vi "Does the Text Fit.vi"(0 "user-specified font":T1, 5 "token string":string, 7 "Capitalize Text":bool) -> (4 "Text Fits":bool)   [LabVIEW 2020, in "Text-Based VI Icon.lvlib"]
uses:
  <vilib>/LabVIEW Icon API/Set Text Icon/Text-Based VI Icon.lvlib
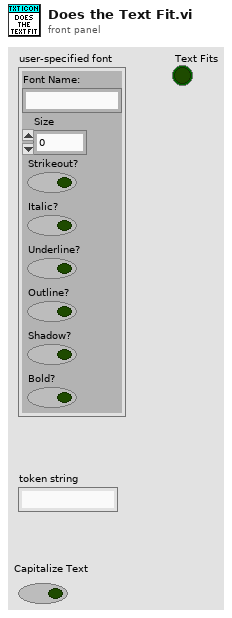
[diagram p1: front panel]
types:
  T1 = cluster{"Font Name:":string, "Size":i16, "Strikeout?":bool, "Italic?":bool, "Underline?":bool, "Outline?":bool, "Shadow?":bool, "Bold?":bool}
  T2 = enum16{"User-specified Font", "Application Font", "System Font", "Dialog Font"}
  T3 = cluster{"left":i16, "top":i16, "right":i16, "bottom":i16}
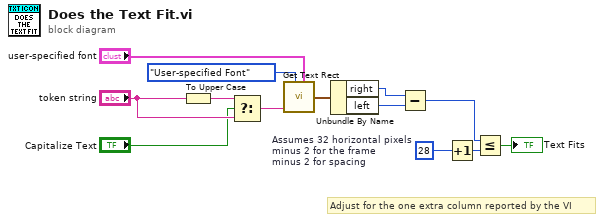
[diagram p0: block diagram]
diagram:
  w9 = i16 28  # Assumes 32 horizontal pixels minus 2 for the frame minus 2 for spacing
  # "Adjust for the one extra column reported by the VI"
  n1 = To Upper Case(1:"token string") -> (0:w4:string)
  n2 = Select(t=w4, s="Capitalize Text", f="token string") -> (s? t:f=w1:string)
  n3 = call <vilib>:"Get Text Rect.vi"("desired font(Application)"=T2."User-specified Font", "text"=w1, "[user-specified font]"="user-specified font") -> ("rect"=w8:T3)  [unwired: 6 in]
  n4 = Unbundle By Name(w8) -> ("right"=w11:i16, "left"=w12:i16)
  n5 = Subtract(x=w11, y=w12) -> (x-y=w13:i16)
  n6 = Increment(x=w9) -> (x+1=w5:i16)
  n7 = Less Or Equal?(x=w13, y=w5) -> (x <= y?=→"Text Fits":bool)
